vi "512bit to 16 IQ samples unpack (14bit).vi"(11 "Element":bool[](array[boolean])) -> (3 "Array":fxp<+/-,14,1>[](array[numeric]))   [LabVIEW 2019, in "FPGA Utility.lvlib"]
uses:
  <instrlib>/_niInstr/Data Formatting/v1/FPGA/Private/Convert/Boolean Array to FXP(+-,14,1) Array.vi
  FPGA Utility.lvlib
  <instrlib>/_niInstr/Data Formatting/v1/FPGA/niInstr Data Formatting v1 FPGA.lvlib
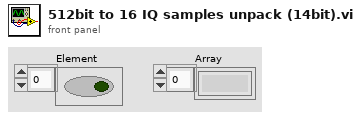
[diagram p1: front panel]
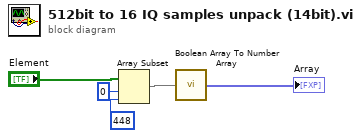
[diagram p0: block diagram]
diagram:
  n1 = Array Subset(array="Element", index=0, length=448) -> (w3:bool[])
  n2 = call-poly <instrlib>:"Boolean Array To Number Array.vi"("data in"=w3) -> ("data out"=→"Array":fxp<+/-,14,1>[])  [unwired: 14 in]
